vi "Calculate Output Impedance.vi"(10 "Current":dbl, 11 "Voltage":dbl) -> (3 "Impedance":dbl)   [LabVIEW 2010]
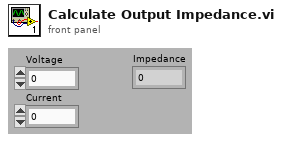
[diagram p1: front panel]
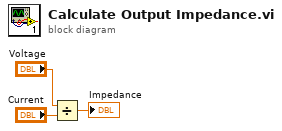
[diagram p0: block diagram]
diagram:
  n1 = Divide(x="Voltage", y="Current") -> (x/y=→"Impedance":dbl)
